vi "Reference GUID Dictionary.vi"(7 "Enum":enum16{"Ref to GUID", "GUID to Ref"}(ring)=enum."GUID to Ref", 8 "error in":errorcluster, 11 "Channel Ref":T1 format="%.0x") -> (0 "error out":errorcluster, 2 "GUID":string, 3 "Channel Ref Out":T1 format="%.0x")   [LabVIEW 2018, in "Instrument Addon Scripting API.lvlib"]
uses:
  Instrument Addon Scripting API.lvlib
  <vilib>/NI Veristand/Custom Device API/Custom Device Item Ref.ctl
  <vilib>/NI VeriStand/Custom Device API/Custom Device API.lvlib
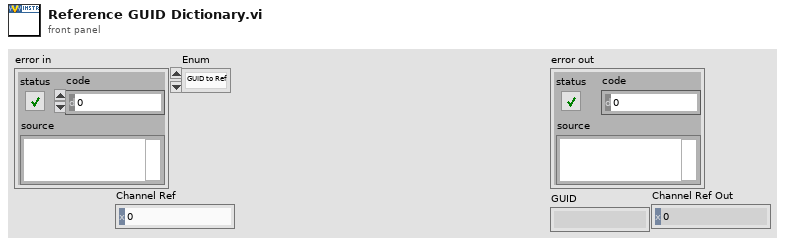
[diagram p1: front panel]
types:
  T1 = typedef "Custom Device API.lvlib/Custom Device Item Ref.ctl" = u64
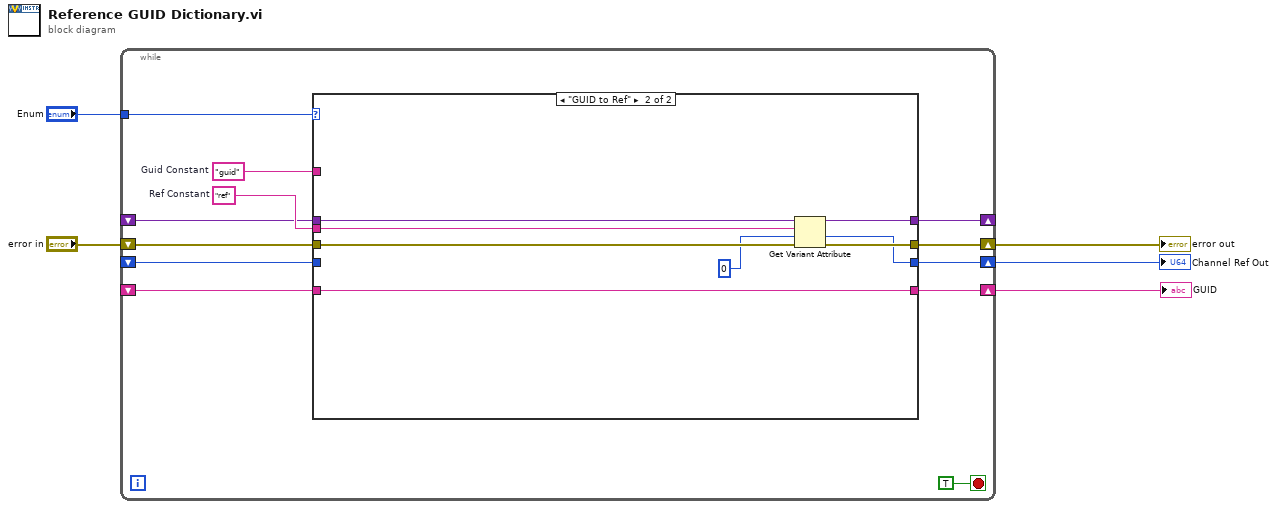
[diagram p0: block diagram]
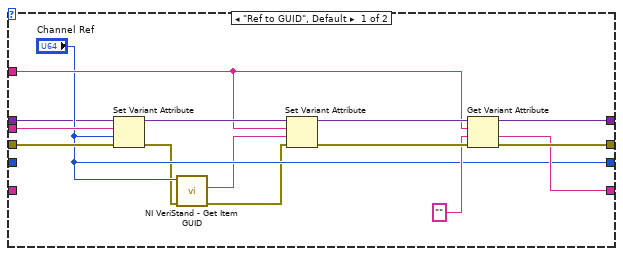
[diagram p2: hidden frame]
diagram:
  n1 = while {
    tunnel: "Enum" -> [w13]
    shift-right: [w11] -> w1
    shift-left: _ -> [w17]
    shift-right: [w15] -> w4
    shift-left: "error in" -> [w16]
    shift-right: [w8] -> w3
    shift-left: _ -> [w12]
    shift-right: [w7] -> _
    shift-left: _ -> [w6]
    stop <- TRUE stop-if-true
    w10 = "guid"  # Guid Constant
    w14 = "ref"  # Ref Constant
    n2 = case shown="\"GUID to Ref\"" w13 {
      tunnel: w6 -> [w18 w40]
      tunnel: w17 -> [_ _]
      tunnel: w16 -> [w31 w39]
      tunnel: [w28 w38] -> w15
      tunnel: w14 -> [w27 w35]
      tunnel: [w25 w33] -> w8
      tunnel: w12 -> [_ w33]
      tunnel: ["Channel Ref" w36] -> w11
      tunnel: w10 -> [w24 _]
      tunnel: [w19 w34] -> w7
      frame "Ref to GUID", Default {
        n3 = Set Variant Attribute(Variant=w18, name=w27, value="Channel Ref", error in=w31) -> (Variant out=w32:variant, error out=w21:errorcluster)  [unwired: 1 out]
        n4 = call <vilib>:"NI VeriStand - Get Item GUID.vi"("error in (no error)"=w21, "Item Ref in"="Channel Ref") -> ("error out"=w20:errorcluster, "GUID"=w22:string)  [unwired: 7 in, 1 out]
        n5 = Set Variant Attribute(Variant=w32, name=w24, value=w22, error in=w20) -> (Variant out=w30:variant, error out=w29:errorcluster)  [unwired: 1 out]
        n6 = Get Variant Attribute(Variant=w30, name=w24, default value (empty Variant)="", error in=w29) -> (duplicate Variant=w19:variant, value=w25:string, error out=w28:errorcluster)  [unwired: 1 out]
      }
      frame "GUID to Ref" {
        n7 = Get Variant Attribute(Variant=w40, name=w35, default value (empty Variant)=T1 0 ("Channel Ref Out"), error in=w39) -> (duplicate Variant=w34:variant, value=w36:T1, error out=w38:errorcluster)  [unwired: 1 out]
      }
    }
  }
  "error out" <- w4
  "GUID" <- w3
  "Channel Ref Out" <- w1
